vi "Result_Test.vi"(8 "error in (no error)":errorcluster caption="entrée d'erreur (pas d'erreur)", 11 "Flash_Jlink en entrée":refnum<class "Get_Install_Code.lvclass">) -> (0 "error out":errorcluster caption="sortie d'erreur", 3 "Flash_Jlink en sortie":refnum<class "Get_Install_Code.lvclass">)   [LabVIEW 2020, in "Library Test.lvlib" / "Get_Install_Code.lvclass"]
uses:
  Get_Install_Code.lvclass
  C:/Users/ngarcin/OneDrive - Altyor/Standard TB/Suite TB45/Class/Test/Test (Default)/Test (Default).lvclass
  Commun VI/TypeDef/Variable Printable.ctl
  Flash_Commander/Flash_Commander.lvclass
  Commun VI/Library Commun.lvlib
panel:
  out "Return_State_Machine (Json)":string
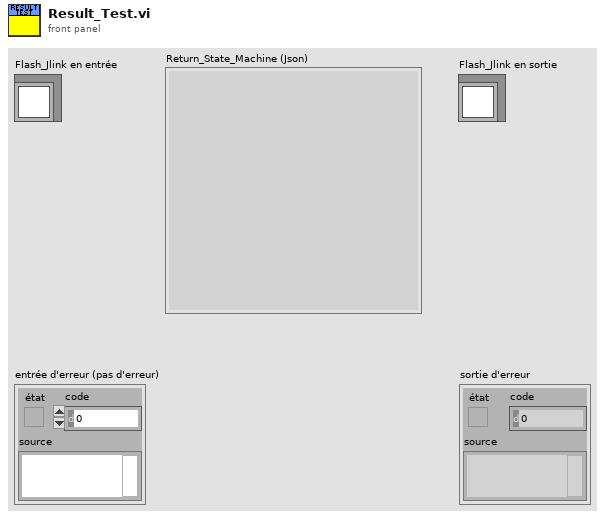
[diagram p1: front panel]
types:
  T1 = typedef "Variable Printable.ctl" = string
  T2 = enum16{"Get Variable", "Get All Variables", "Set Variable", "Delete Variable", "Delete All Variable"}
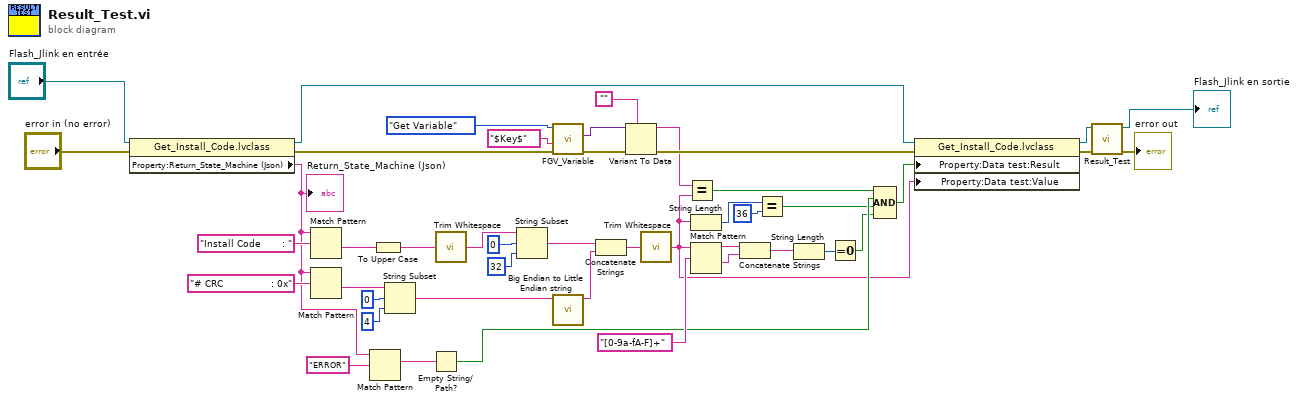
[diagram p0: block diagram]
diagram:
  n1 = property class="Get_Install_Code.lvclass"(reference="Flash_Jlink en entrée", error in="error in (no error)") -> (reference out=w28:refnum<class "Get_Install_Code.lvclass">, error out=w24:errorcluster, "Property:Return_State_Machine (Json)"=w13:string)
  "Return_State_Machine (Json)" <- w13
  n2 = Match Pattern(string=w13, regular expression="Install Code       : ") -> (after substring=w22:string)  [unwired: 1 in, 3 out]
  n3 = Match Pattern(string=w13, regular expression="# CRC                : 0x" ("chaîne")) -> (after substring=w10:string)  [unwired: 1 in, 3 out]
  n4 = Match Pattern(string=w13, regular expression="ERROR" ("expression régulière")) -> (match substring=w45:string)  [unwired: 1 in, 3 out]
  n5 = To Upper Case(1:w22) -> (0:w43:string)
  n6 = String Subset(string=w10, offset (0)=0 ("length (rest)"), length (rest)=4 ("length (rest)")) -> (substring=w9:string)
  n7 = Empty String/Path?(string/path=w45) -> (empty?=w31:bool)
  n8 = call <vilib>:"Trim Whitespace.vi"("string"=w43) -> ("trimmed string"=w39:string)  [unwired: 1 in]
  n9 = String Subset(string=w39, offset (0)=0 ("length (rest)"), length (rest)=32 ("length (rest)")) -> (substring=w12:string)
  n10 = call "FGV_Variable.vi"("error in (no error)"=w24, "Variable"=T1 "$Key$" ("Variable Printable"), "Function"=T2."Get Variable") -> ("error out"=w23:errorcluster, "Data Out"=w20:variant)  [unwired: 6 in, 1 out]
  n11 = call "Big Endian to Little Endian string.vi"("Input (Big Endian)"=w9) -> ("Output (Little Endian)"=w8:string)  [unwired: 10 in]
  n12 = Concatenate Strings(w12, w8) -> (w11:string)
  n13 = Variant To Data(error in=w23, type="", Variant=w20) -> (data=w18:string, error out=w21:errorcluster)
  n14 = call <vilib>:"Trim Whitespace.vi"("string"=w11) -> ("trimmed string"=w7:string)  [unwired: 1 in]
  n15 = Equal?(x=w18, y=w7) -> (x = y?=w17:bool)
  n16 = String Length(string=w7) -> (length=w32:i32)
  n17 = Match Pattern(string=w7, regular expression="[0-9a-fA-F]+") -> (before substring=w33:string, after substring=w34:string)  [unwired: 1 in, 2 out]
  n18 = Concatenate Strings(w33, w34) -> (w35:string)
  n19 = Equal?(x=w32, y=36) -> (x = y?=w30:bool)
  n20 = String Length(string=w35) -> (length=w36:i32)
  n21 = Equal To 0?(x=w36) -> (x = 0?=w29:bool)
  n22 = Compound Arithmetic op=AND(w17, w31, w30, w29) -> (w27:bool)
  n23 = property class="Get_Install_Code.lvclass"(reference=w28, error in=w21, "Property:Data test:Result"=w27, "Property:Data test:Value"=w7) -> (reference out=w3:refnum<class "Get_Install_Code.lvclass">, error out=w6:errorcluster)
  n24 = call-parent "Result_Test.vi"("error in (no error)"=w6, "Flash_Jlink en entrée"=w3) -> ("error out"=→"error out":errorcluster, "Flash_Jlink en sortie"=→"Flash_Jlink en sortie":refnum<class "Get_Install_Code.lvclass">)  [unwired: 8 in]
